vi "Destroy to SSH.vi"(8 "Error In":errorcluster, 11 "Identity":refnum<class "Agent Identity.lvclass">) -> (0 "Error Out":errorcluster, 3 "SSH":refnum<class "SSH.lvclass">)   [LabVIEW 2018, in "Toolkit.lvlib" / "Agent Identity.lvclass"]
doc: "Deallocates, or frees, the memory allocated for the agent identity object. The identity object cannot be used after it is destroyed; otherwise, a segmentation fault will occur."
uses:
  Agent Identity.lvclass
  SSH/SSH.lvclass
  Agent Identity.lvclass/Agent Identity.ctl
  SSH/SSH.lvclass/SSH.ctl
  Toolkit.lvlib
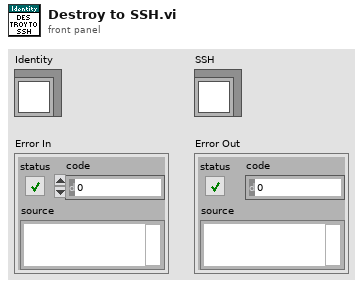
[diagram p1: front panel]
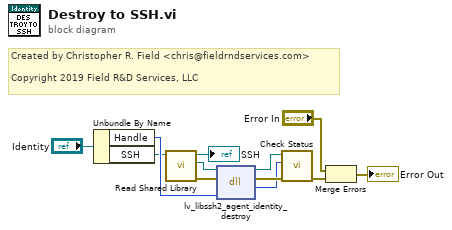
[diagram p0: block diagram]
diagram:
  # "Created by Christopher R. Field <chris@fieldrndservices.com>\n\nCopyright 2019 Field R&D Services, LLC"
  n1 = Unbundle By Name("Identity") -> ("Handle"=w10:u64, "SSH"=w5:refnum<class "SSH.lvclass">)
  n2 = call "Read Shared Library.vi"("SSH In"=w5) -> ("Error Out"=w4:errorcluster, "lv-libssh2 Shared Library"=w3:path, "SSH Out"=→"SSH":refnum<class "SSH.lvclass">)  [unwired: 8 in]
  n3 = dll-call lib="lv-libssh2.*" fn="lv_libssh2_agent_identity_destroy"(path in=w3, error in=w4, "handle"=w10) -> (path out=w8:path, error out=w9:errorcluster, "status"=w7:i32)  [unwired: 2 in]
  n4 = call "Check Status.vi"("Error In"=w9, "Status"=w7, "lv-libssh2 Shared Library In"=w8) -> ("Error Out"=w6:errorcluster)  [unwired: 7 in, 1 out]
  n5 = Merge Errors("Error In", w6) -> (→"Error Out":errorcluster)
